vi "Instrument Manager Loop.vi"(8 "System Control":refnum<queue>, 11 "Instrument Manager":refnum<queue>) -> (0 "error out":errorcluster)   [LabVIEW 2020, in "Mock Pump Controller.lvlib" / "Instrument Manager.lvlib"]
uses:
  Instrument Manager/Instrument Manager.lvlib
  support/Message Queue/Message Cluster.ctl
  Instrument Manager/Instrument State.ctl
  <vilib>/Utility/error.llb/Error Cluster From Error Code.vi
  <vilib>/ErrorRing/Error Ring.xnode
  Mock Pump Controller.lvlib
  support/Message Queue/Message Queue.lvlib
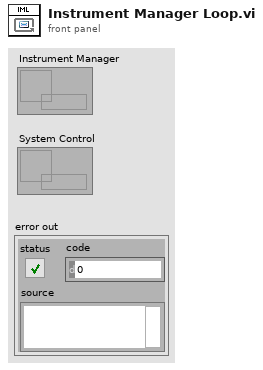
[diagram p1: front panel]
types:
  T1 = typedef "Mock Pump Controller.lvlib/Instrument Manager.lvlib/Instrument State.ctl" = cluster{"VISA Resource":refnum<visa-resource-name>, "Flow Rate":dbl, "Running":bool, "Running Since":timestamp, "Pressure Data Point":cluster{"Time Stamp":timestamp, "Value":dbl}, "Upper Pressure Fault":bool, "Lower Pressure Fault":bool, "Motor Stall Fault":bool, "Sampling Rate (sec/sample)":dbl}
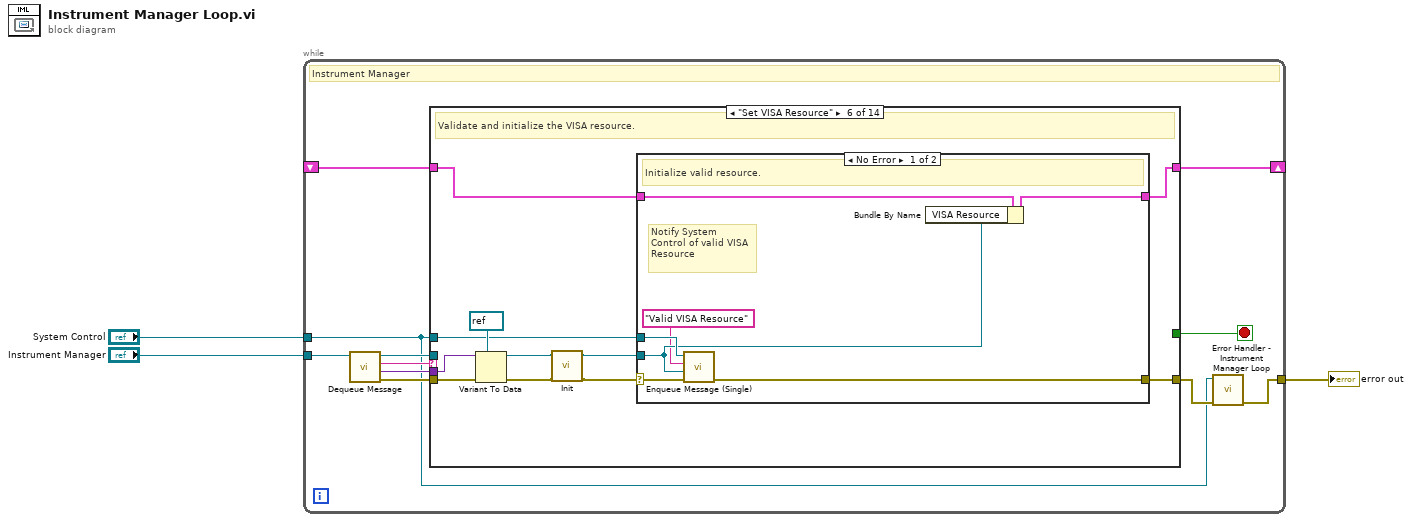
[diagram p0: block diagram]
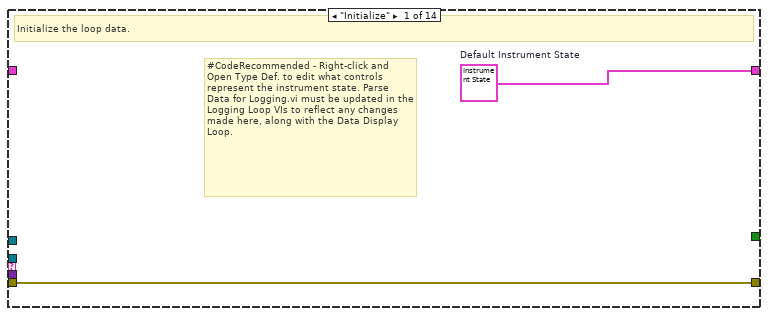
[diagram p2: hidden frame]
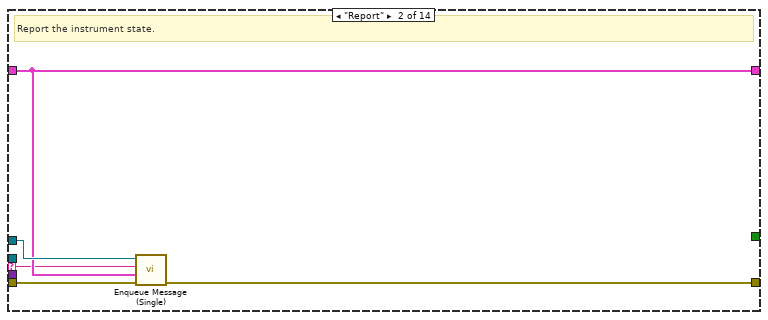
[diagram p3: hidden frame]
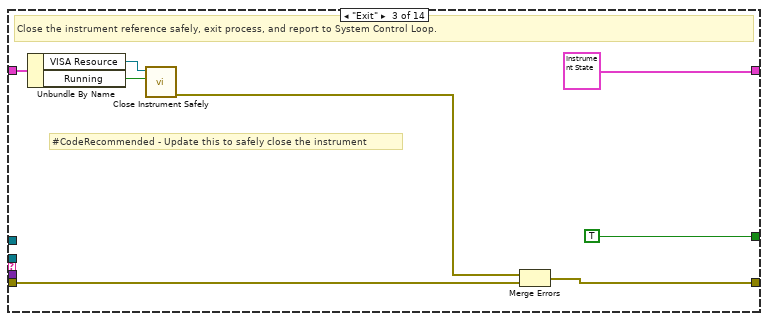
[diagram p4: hidden frame]
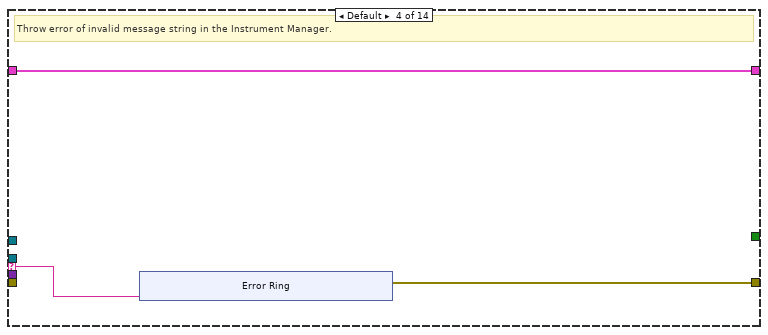
[diagram p5: hidden frame]
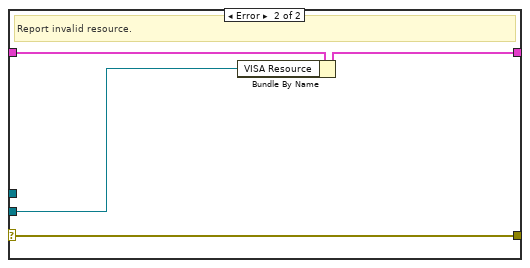
[diagram p7: hidden frame]
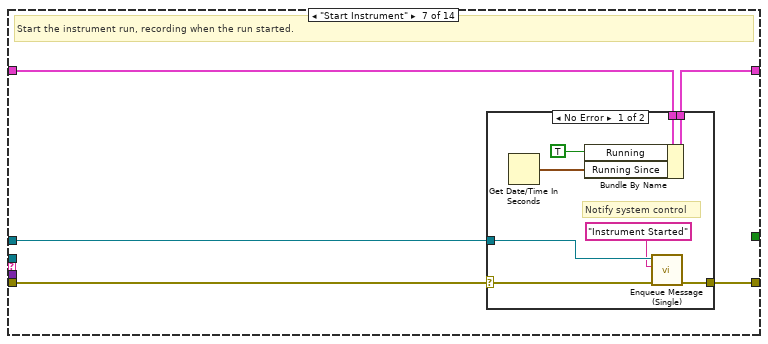
[diagram p8: hidden frame]
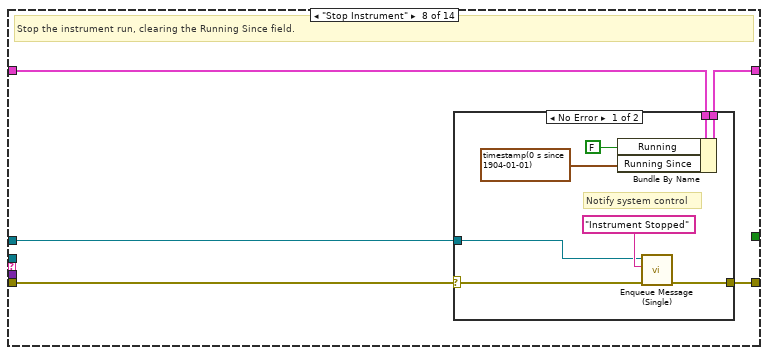
[diagram p10: hidden frame]
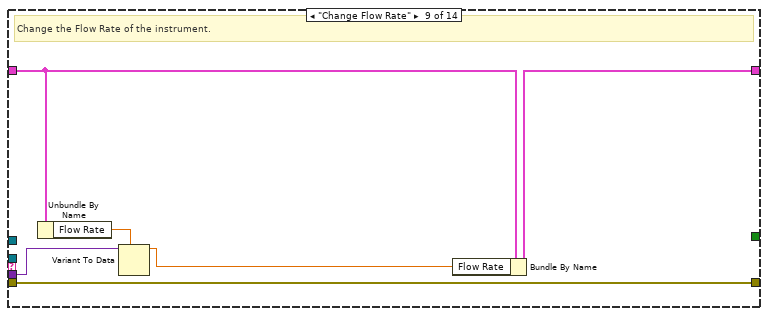
[diagram p12: hidden frame]
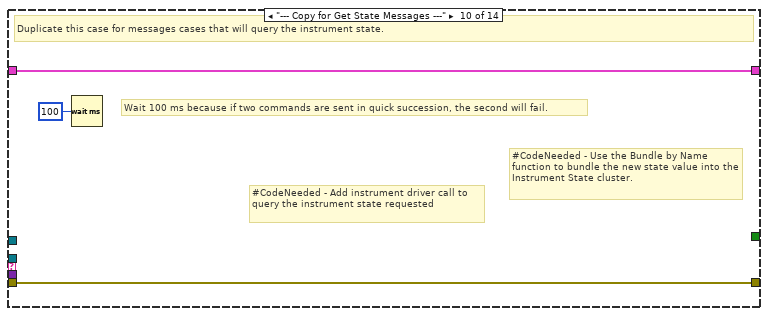
[diagram p13: hidden frame]
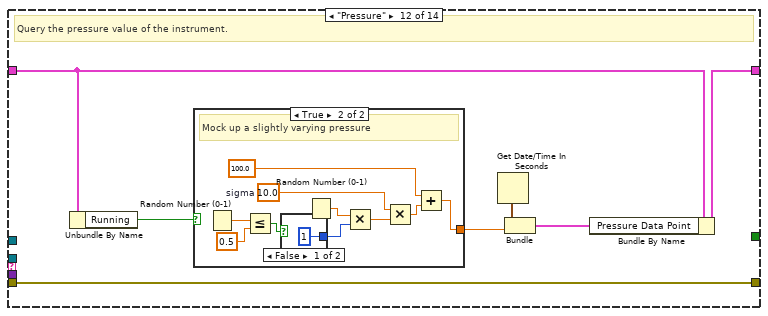
[diagram p15: hidden frame]
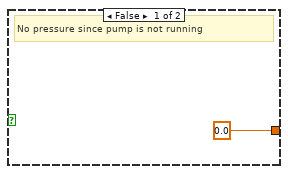
[diagram p16: hidden frame]
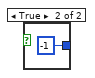
[diagram p17: hidden frame]
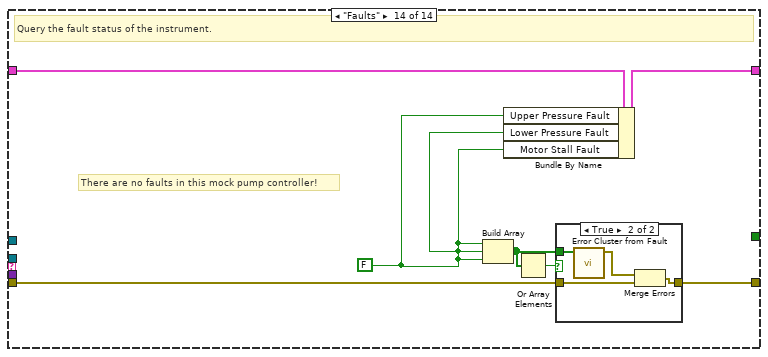
[diagram p19: hidden frame]
diagram:
  n1 = while {
    tunnel: "Instrument Manager" -> [w14]
    tunnel: "System Control" -> [w4]
    tunnel: [w8] -> w1
    shift-right: [w6] -> _
    shift-left: _ -> [w7]
    stop <- w5 stop-if-true
    # "Instrument Manager"
    n2 = call "Dequeue Message.vi"("Message Queue"=w14) -> ("error out"=w10:errorcluster, "Message Data"=w11:variant, "Message"=w13:string, "dup Message Queue"=w12:refnum<queue>)  [unwired: 7 in]
    n3 = case shown="\"Set VISA Resource\"" w13 {
      selector: w13 -> [_ w17 _ w31 _ _ _ _ _ _ _ _ _ _]
      tunnel: w12 -> [_ _ _ _ _ _ _ _ _ _ _ _ _ _]
      tunnel: w4 -> [_ w20 _ _ _ w46 w67 w82 _ _ _ _ _ _]
      tunnel: w11 -> [_ _ _ _ _ w49 _ _ w98 _ _ _ _ _]
      tunnel: w10 -> [w15 w21 w24 _ w40 w48 w65 w80 w94 w102 w104 w108 w126 w128]
      tunnel: [w15 w19 w23 w30 w40 w52 w68 w83 w94 w102 w104 w108 w126 w131] -> w9
      tunnel: w7 -> [_ w18 w29 w32 w41 w51 w64 w79 w97 w101 w103 w106 w125 w132]
      tunnel: [w16 w18 T1 {"VISA Resource"="", "Flow Rate"=0.0, "Running"=FALSE, "Running Since"=timestamp(0 s since 1904-01-01), "Pressure Data Point"={"Time Stamp"=timestamp(0 s since 1904-01-01), "Value"=0.0}, "Upper Pressure Fault"=FALSE, "Lower Pressure Fault"=FALSE, "Motor Stall Fault"=FALSE, "Sampling Rate (sec/sample)"=0.0} w32 w41 w50 w66 w81 w99 w101 w103 w111 w125 w133] -> w6
      tunnel: [_ _ TRUE _ _ _ _ _ _ _ _ _ _ _] -> w5
      frame "Initialize" {
        w16 = T1 {"VISA Resource"="", "Flow Rate"=0.0, "Running"=FALSE, "Running Since"=timestamp(0 s since 1904-01-01), "Pressure Data Point"={"Time Stamp"=timestamp(0 s since 1904-01-01), "Value"=0.0}, "Upper Pressure Fault"=FALSE, "Lower Pressure Fault"=FALSE, "Motor Stall Fault"=FALSE, "Sampling Rate (sec/sample)"=0.0}  # Default Instrument State
        # "#CodeRecommended - Right-click and Open Type Def. to edit what controls represent the instrument state. Parse Data for Logging.vi must be updated in the Logging Loop VIs to reflect any changes made here, along with the Data Display Loop."
        # "Initialize the loop data."
      }
      frame "Report" {
        # "Report the instrument state."
        n4 = call "Enqueue Message (Single).vi"("error in (no error)"=w21, "Message Data"=w18, "Message"=w17, "Message Queue"=w20) -> ("error out"=w19:errorcluster)  [unwired: 6 in, 1 out]
      }
      frame "Exit" {
        # "#CodeRecommended - Update this to safely close the instrument"
        # "Close the instrument reference safely, exit process, and report to System Control Loop."
        n5 = Unbundle By Name(w29) -> ("VISA Resource"=w27:refnum<visa-resource-name>, "Running"=w28:bool)
        n6 = call "Close Instrument Safely.vi"("Running (F)"=w28, "VISA Refnum in"=w27) -> ("error out"=w22:errorcluster)  [unwired: 9 in]
        n7 = Merge Errors(w22, w24) -> (w23:errorcluster)
      }
      frame Default {
        # "Throw error of invalid message string in the Instrument Manager."
        n8 = xnode "Error Ring"("parameter 0"=w31) -> ("error out"=w30:errorcluster)
      }
      frame "--- Copy This Frame ---" {
        # "Copy this frame and add responses to instrument specific messages."
      }
      frame "Set VISA Resource" {
        # "Validate and initialize the VISA resource."
        n9 = Variant To Data(error in=w48, type=refnum<visa-resource-name> refnum, Variant=w49) -> (data=w43:refnum<visa-resource-name>, error out=w42:errorcluster)
        n10 = call "Init.vi"("error in (no error)"=w42, "VISA resource name"=w43) -> ("error out"=w45:errorcluster, "VISA resource out"=w44:refnum<visa-resource-name>)  [unwired: 8 in]
        n11 = case shown="No Error" w45 {
          selector: w45 -> [w58 w60]
          tunnel: w44 -> [w55 w61]
          tunnel: [w57 w60] -> w52
          tunnel: w51 -> [w59 w63]
          tunnel: [w53 w62] -> w50
          tunnel: w46 -> [w56 _]
          frame No Error {
            # "Notify System Control of valid VISA Resource"
            # "Initialize valid resource."
            n12 = call "Enqueue Message (Single).vi"("error in (no error)"=w58, "Message Data"=w55, "Message"="Valid VISA Resource", "Message Queue"=w56) -> ("error out"=w57:errorcluster)  [unwired: 6 in, 1 out]
            n13 = Bundle By Name(cluster=w59, "VISA Resource"=w55) -> (w53:T1)
          }
          frame Error {
            # "Report invalid resource."
            n14 = Bundle By Name(cluster=w63, "VISA Resource"=w61) -> (w62:T1)
          }
        }
      }
      frame "Start Instrument" {
        # "Start the instrument run, recording when the run started."
        n15 = case shown="No Error" w65 {
          selector: w65 -> [w69 w78]
          tunnel: [w76 w78] -> w68
          tunnel: w67 -> [w75 _]
          tunnel: [w73 w77] -> w66
          tunnel: w64 -> [w70 w77]
          frame No Error {
            # "Notify system control"
            n16 = Get Date/Time In Seconds() -> (seconds since 1Jan1904=w71:timestamp)
            n17 = Bundle By Name(cluster=w70, "Running"=TRUE, "Running Since"=w71) -> (w73:T1)
            n18 = call "Enqueue Message (Single).vi"("error in (no error)"=w69, "Message"="Instrument Started", "Message Queue"=w75) -> ("error out"=w76:errorcluster)  [unwired: 7 in, 1 out]
          }
          frame Error {
          }
        }
      }
      frame "Stop Instrument" {
        # "Stop the instrument run, clearing the Running Since field."
        n19 = case shown="No Error" w80 {
          selector: w80 -> [w84 w93]
          tunnel: w79 -> [w91 w92]
          tunnel: [w90 w93] -> w83
          tunnel: w82 -> [w88 _]
          tunnel: [w87 w92] -> w81
          frame No Error {
            # "Notify system control"
            n20 = Bundle By Name(cluster=w91, "Running"=FALSE, "Running Since"=timestamp(0 s since 1904-01-01)) -> (w87:T1)
            n21 = call "Enqueue Message (Single).vi"("error in (no error)"=w84, "Message"="Instrument Stopped", "Message Queue"=w88) -> ("error out"=w90:errorcluster)  [unwired: 7 in, 1 out]
          }
          frame Error {
          }
        }
      }
      frame "Change Flow Rate" {
        # "Change the Flow Rate of the instrument."
        n22 = Unbundle By Name(w97) -> ("Flow Rate"=w96:dbl)
        n23 = Variant To Data(type=w96, Variant=w98) -> (data=w95:dbl)  [unwired: 1 in, 1 out]
        n24 = Bundle By Name(cluster=w97, "Flow Rate"=w95) -> (w99:T1)
      }
      frame "--- Copy for Get State Messages ---" {
        # "Wait 100 ms because if two commands are sent in quick succession, the second will fail."
        # "#CodeNeeded - Use the Bundle by Name function to bundle the new state value into the Instrument State cluster."
        # "#CodeNeeded - Add instrument driver call to query the instrument state requested"
        # "Duplicate this case for messages cases that will query the instrument state."
        n25 = Wait (ms)(milliseconds to wait=u32 100) -> ()  [unwired: 1 out]
      }
      frame "Run State" {
        # "Since this is a mock pump, no query is necessary here"
        # "Query the run state of the instrument."
      }
      frame "Pressure" {
        # "Query the pressure value of the instrument."
        n26 = Unbundle By Name(w106) -> ("Running"=w105:bool)
        n27 = case shown="True" w105 {
          tunnel: [0.0 w118] -> w107
          frame False {
            # "No pressure since pump is not running"
          }
          frame True {
            w120 = 10.0  # sigma
            # "Mock up a slightly varying pressure"
            n28 = Random Number (0-1)() -> (number: 0 to 1=w122:dbl)
            n29 = Less Or Equal?(x=w122, y=0.5) -> (x <= y?=w113:bool)
            n30 = case shown="False" w113 {
              tunnel: [1 -1] -> w117
              frame False {
              }
              frame True {
              }
            }
            n31 = Random Number (0-1)() -> (number: 0 to 1=w116:dbl)
            n32 = Multiply(x=w116, y=w117) -> (x*y=w115:dbl)
            n33 = Multiply(x=w120, y=w115) -> (x*y=w114:dbl)
            n34 = Add(x=100.0, y=w114) -> (x+y=w118:dbl)
          }
        }
        n35 = Get Date/Time In Seconds() -> (seconds since 1Jan1904=w110:timestamp)
        n36 = Bundle("seconds since 1Jan1904"=w110, w107) -> (w109:cluster{"seconds since 1Jan1904":timestamp, dbl})  [unwired: 1 in]
        n37 = Bundle By Name(cluster=w106, "Pressure Data Point"=w109) -> (w111:T1)
      }
      frame "Flow Rate" {
        # "Mock pump, so no queries are necessary"
        # "Query the flow rate of the instrument."
      }
      frame "Faults" {
        w127 = FALSE
        # "There are no faults in this mock pump controller!"
        # "Query the fault status of the instrument."
        n38 = Build Array(w127, w127, w127) -> (w129:bool[])
        n39 = Bundle By Name(cluster=w132, "Upper Pressure Fault"=w127, "Lower Pressure Fault"=w127, "Motor Stall Fault"=w127) -> (w133:T1)
        n40 = Or Array Elements(Boolean array=w129) -> (logical OR=w130:bool)
        n41 = case shown="True" w130 {
          tunnel: w128 -> [w134 w138]
          tunnel: [w134 w137] -> w131
          tunnel: w129 -> [_ w135]
          frame False {
          }
          frame True {
            n42 = call "Error Cluster from Fault.vi"("Fault indicators"=w135) -> ("error out"=w136:errorcluster)  [unwired: 10 in]
            n43 = Merge Errors(w136, w138) -> (w137:errorcluster)
          }
        }
      }
    }
    n44 = call "Error Handler - Instrument Manager Loop.vi"("error in (no error)"=w9, "Message Queue"=w4) -> ("dup error in"=w8:errorcluster)  [unwired: 8 in, 1 out]
  }
  "error out" <- w1
